vi "Motor controller.vi"() -> ()   [LabVIEW 2012]
uses:
  BotStatus.vi
  <vilib>/Rock Robotics/WPI/Solenoid/WPI_SolenoidSetEnum.vi
  <vilib>/Rock Robotics/WPI/Solenoid/WPI_SolenoidValue.ctl
panel:
  out "Transferable":bool
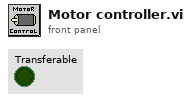
[diagram p1: front panel]
types:
  T1 = typedef "WPI_SolenoidValue.ctl" = enum16{"Off", "On", "Forward", "Reverse"}
  T2 = typedef "WPI_MotorControlDeviceRef.ctl" = cluster{"DeviceStatus":errorcluster, "Type":enum16{"PWM", "CAN"}, "PWM":cluster{"Digital Module":T3, "PWM Channel":T4, "DeadBand":T5}, "CAN":cluster{"Device Number":u8, "Control Mode":T6, "Semaphore":T7, "Max Vout":dbl}, "Invert":bool, "TransformRef":T8, "InvTransformRef":T8}
  T3 = typedef "FPGA_TypedefDigitalModule.ctl" = enum16{"Digital Module 1", "Digital Module 2"}
  T4 = typedef "FPGA_DIOPWMChannel.ctl" = enum8{"PWM 1", "PWM 2", "PWM 3", "PWM 4", "PWM 5", "PWM 6", "PWM 7", "PWM 8", "PWM 9", "PWM 10", "Invalid"}
  T5 = typedef "WPI_PWMDeadband.ctl" = cluster{"Name":string, "maxPositivePwm":i32, "minPositivePwm":i32, "centerPwm":i32, "maxNegativePwm":i32, "minNegativePwm":i32, "angularRange":u16}
  T6 = typedef "WPI_CANJaguar_ControlMode.ctl" = enum8{"Percent VBus", "Current", "Speed", "Position", "Voltage"}
  T7 = typedef "Semaphore RefNum" = refnum<k1>
  T8 = typedef "WPI_PWMTransform_ConPane.ctl" = refnum<vi>
  T9 = typedef "WPI_EncoderDevRef.ctl" = cluster{"DevStatus":errorcluster, "EncoderIndex":T10, "CounterIndex":T11, "DistancePerCount":dbl, "Decoding Type":T12}
  T10 = typedef "FPGA_EncoderIdx.ctl" = enum8{"Enc 0", "Enc 1", "Enc 2", "Enc 3", "Invalid"}
  T11 = typedef "FPGA_CounterCtrSystemIndex.ctl" = enum8{"Ctr 0", "Ctr 1", "Ctr 2", "Ctr 3", "Ctr 4", "Ctr 5", "Ctr 6", "Ctr 7", "Invalid"}
  T12 = typedef "WPI_EncoderType.ctl" = enum16{"1x", "2x", "4x"}
  T13 = typedef "WPI_RelayDevRef.ctl" = cluster{"DevStatus":errorcluster, "Relay Channel":T14, "Digital Module":T3, "Relay Direction":T15}
  T14 = typedef "FPGA_DIORelayChannel.ctl" = enum8{"Relay 1", "Relay 2", "Relay 3", "Relay 4", "Relay 5", "Relay 6", "Relay 7", "Relay 8", "Invalid"}
  T15 = typedef "WPI_RelayDirection.ctl" = enum16{"Both directions", "Forward only", "Reverse only"}
  T16 = typedef "WPI_RelayValue.ctl" = enum16{"Off", "On", "Forward", "Reverse"}
  T17 = typedef "WPI_ServoDeviceRef.ctl" = cluster{"DeviceStatus":errorcluster, "Digital Module":T3, "PWM Channel":T4, "DeadBand":T5}
  T18 = typedef "WPI_SolenoidDevRef.ctl" = cluster{"DevStatus":errorcluster, "Solenoid Module":T19, "Forward Solenoid Channel":T20, "Reverse Solenoid Channel":T20}
  T19 = typedef "FPGA_TypedefSolenoidModule.ctl" = enum16{"Solenoid Module 1", "Solenoid Module 2"}
  T20 = typedef "WPI_SolenoidChannel.ctl" = enum8{"Solenoid 1", "Solenoid 2", "Solenoid 3", "Solenoid 4", "Solenoid 5", "Solenoid 6", "Solenoid 7", "Solenoid 8", "Invalid"}
  T21 = cluster{"Cannon Upper LS":bool, "Cannon Lower LS":bool}
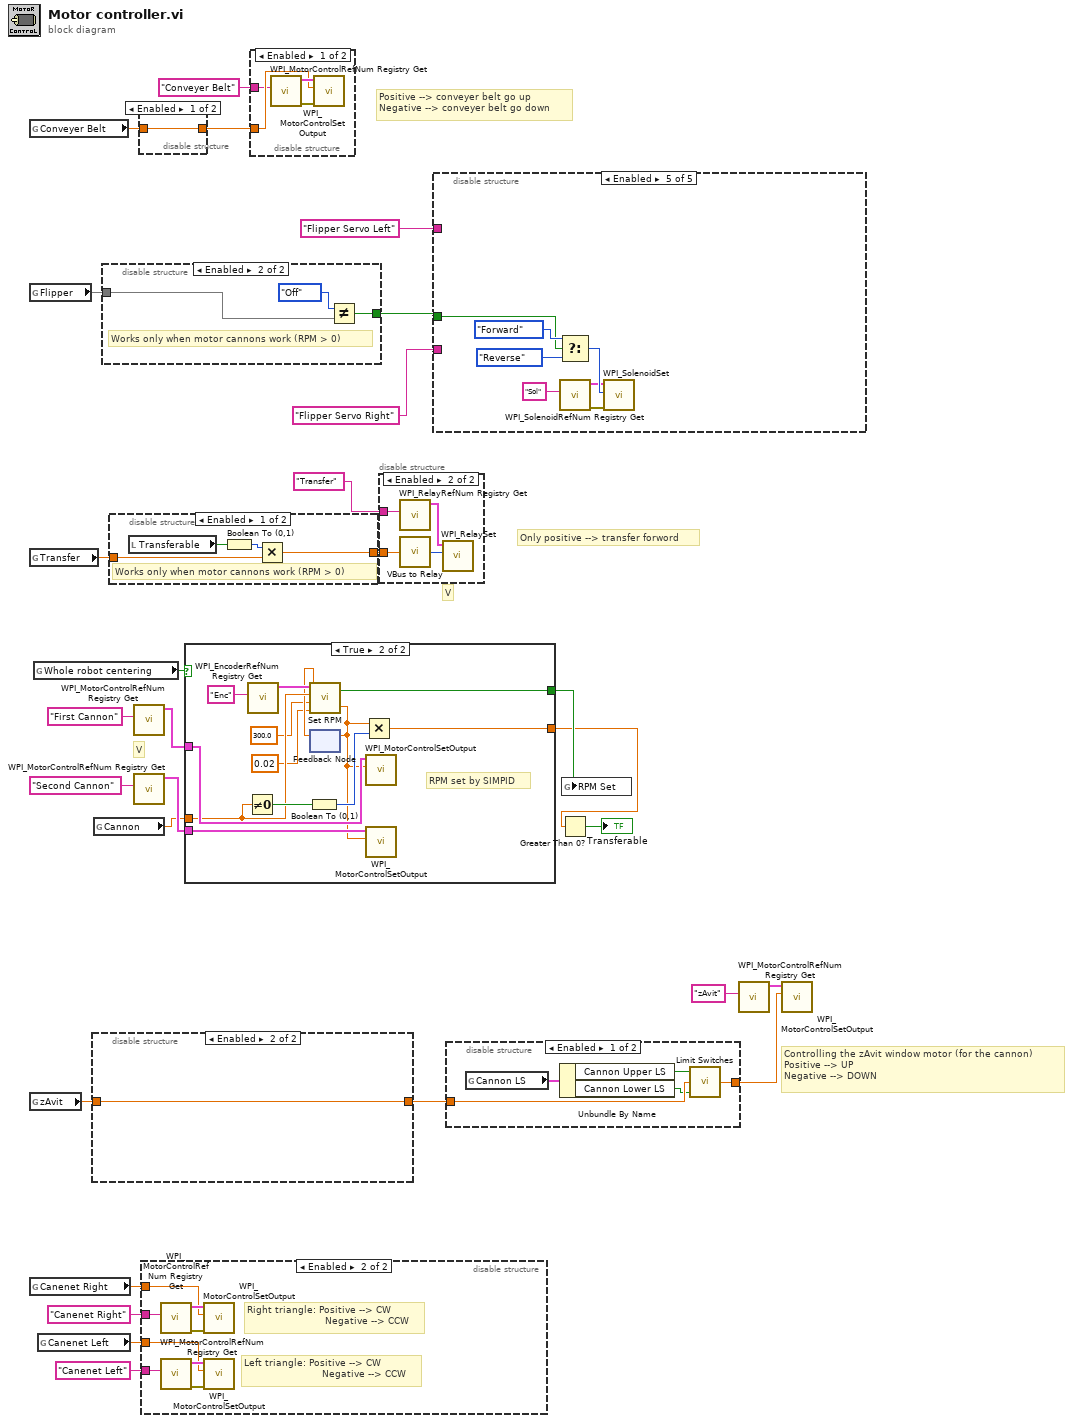
[diagram p0: block diagram]
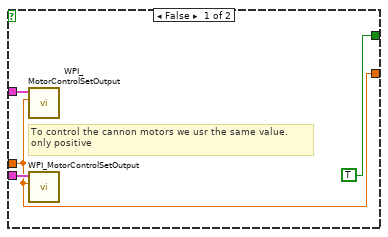
[diagram p2: hidden frame]
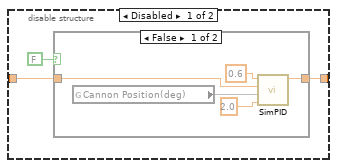
[diagram p4: hidden frame]
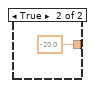
[diagram p5: hidden frame]
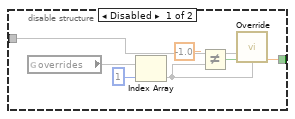
[diagram p8: hidden frame]
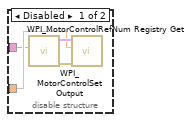
[diagram p10: hidden frame]
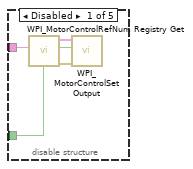
[diagram p11: hidden frame]
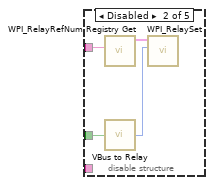
[diagram p12: hidden frame]
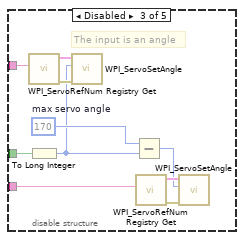
[diagram p13: hidden frame]
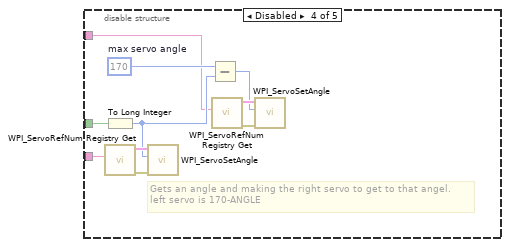
[diagram p14: hidden frame]
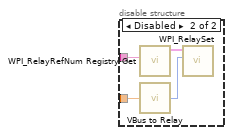
[diagram p15: hidden frame]
diagram:
  # "Positive --> conveyer belt go up\nNegative --> conveyer belt go down"
  # "Only positive --> transfer forword"
  # "Controlling the zAvit window motor (for the cannon)\nPositive --> UP\nNegative --> DOWN"
  # "V"
  # "V"
  n1 = global read "BotStatus.vi" "Conveyer Belt"() -> (w12:dbl)
  n2 = global read "BotStatus.vi" "Flipper"() -> (w13)
  n3 = global read "BotStatus.vi" "Transfer"() -> (w14:dbl)
  n4 = global read "BotStatus.vi" "zAvit"() -> (w15:dbl)
  n5 = global read "BotStatus.vi" "Canenet Right"() -> (w10:dbl)
  n6 = global read "BotStatus.vi" "Whole robot centering"() -> (w1:bool)
  n7 = global read "BotStatus.vi" "Canenet Left"() -> (w11:dbl)
  n8 = disable-structure shown="Enabled" {
    disable-tunnel: [w31 w38] -> w17
    disable-tunnel: w15 -> [w30 w38]
    frame Disabled {
      n9 = case shown="False" FALSE {
        tunnel: [w32 -20.0 ("zAvit")] -> w31
        tunnel: w30 -> [w36 _]
        frame False {
          n10 = global read "BotStatus.vi" "Cannon Position(deg)"() -> (w35)
          n11 = call "SimPID.vi"("Range"=2.0, "Position"=w35, "Set Point"=w36, "Gain"=0.6) -> ("result"=w32:dbl)  [unwired: 5 in, 1 out]
        }
        frame True {
        }
      }
    }
    frame Enabled {
    }
  }
  n12 = global read "BotStatus.vi" "Cannon"() -> (w3:dbl)
  n13 = disable-structure shown="Enabled" {
    disable-tunnel: w13 -> [w45 w48]
    disable-tunnel: [w44 w47] -> w19
    frame Disabled {
      n14 = global read "BotStatus.vi" "overrides"() -> (w43)
      n15 = Index Array(array=w43, index=1) -> (element=w39)
      n16 = Not Equal?(x=-1.0, y=w39) -> (x != y?=w40:bool)
      n17 = call "Override.vi"("Regualer"=w45, "Override"=w40, "Overriden"=w39) -> ("Output"=w44:dbl)  [unwired: 12 in]
    }
    frame Enabled {
      # "Works only when motor cannons work (RPM > 0)"
      n18 = Not Equal?(x=WPI_SolenoidValue."Off" ("Value"), y=w48) -> (x != y?=w47:bool)
    }
  }
  n19 = disable-structure shown="Enabled" {
    disable-tunnel: w14 -> [w52 w53]
    disable-tunnel: [w49 w53] -> w18
    frame Enabled {
      # "Works only when motor cannons work (RPM > 0)"
      n20 = local read "Transferable"() -> (w51:bool)
      n21 = Boolean To (0,1)(Boolean=w51) -> (0, 1=w50:i16)
      n22 = Multiply(x=w50, y=w52) -> (x*y=w49:dbl)
    }
    frame Disabled {
    }
  }
  n23 = call <vilib>:"WPI_MotorControlRefNum Registry Get.vi"("refnum name"="First Cannon") -> ("MotorControlDevRef"=w7:T2)  [unwired: 9 in, 1 out]
  n24 = call <vilib>:"WPI_MotorControlRefNum Registry Get.vi"("refnum name"="Second Cannon") -> ("MotorControlDevRef"=w6:T2)  [unwired: 9 in, 1 out]
  n25 = disable-structure shown="Enabled" {
    disable-tunnel: [w54 w55] -> w20
    disable-tunnel: w12 -> [w54 w55]
    frame Enabled {
    }
    frame Disabled {
    }
  }
  n26 = disable-structure shown="Enabled" {
    disable-tunnel: "Canenet Right" ("refnum name") -> [_ w59]
    disable-tunnel: "Canenet Left" ("refnum name") -> [_ w58]
    disable-tunnel: w10 -> [_ w57]
    disable-tunnel: w11 -> [_ w56]
    frame Disabled {
    }
    frame Enabled {
      # "Left triangle: Positive --> CW\n                          Negative --> CCW"
      # "Right triangle: Positive --> CW\n                          Negative --> CCW"
      n27 = call <vilib>:"WPI_MotorControlRefNum Registry Get.vi"("refnum name"=w59) -> ("error out"=w63:errorcluster, "MotorControlDevRef"=w62:T2)  [unwired: 9 in]
      n28 = call <vilib>:"WPI_MotorControlRefNum Registry Get.vi"("refnum name"=w58) -> ("error out"=w60:errorcluster, "MotorControlDevRef"=w61:T2)  [unwired: 9 in]
      n29 = call <vilib>:"WPI_MotorControlSetOutput.vi"("error in (no error)"=w63, "Output"=w57, "MotorControlDevRef"=w62) -> ()  [unwired: 6 in, 3 out]
      n30 = call <vilib>:"WPI_MotorControlSetOutput.vi"("error in (no error)"=w60, "Output"=w56, "MotorControlDevRef"=w61) -> ()  [unwired: 6 in, 3 out]
    }
  }
  n31 = case shown="True" w1 {
    tunnel: w7 -> [w67 w76]
    tunnel: w6 -> [w66 w75]
    tunnel: [TRUE w74] -> w4
    tunnel: w3 -> [w64 w72]
    tunnel: [w64 w73] -> w2
    frame False {
      # "To control the cannon motors we usr the same value.\nonly positive"
      n32 = call <vilib>:"WPI_MotorControlSetOutput.vi"("Output"=w64, "MotorControlDevRef"=w67) -> ()  [unwired: 7 in, 3 out]
      n33 = call <vilib>:"WPI_MotorControlSetOutput.vi"("Output"=w64, "MotorControlDevRef"=w66) -> ()  [unwired: 7 in, 3 out]
    }
    frame True {
      # "RPM set by SIMPID"
      n34 = Not Equal To 0?(x=w72) -> (x != 0?=w78:bool)
      n35 = call <vilib>:"WPI_EncoderRefNum Registry Get.vi"("refnum name"="Enc") -> ("EncoderDevRef"=w79:T9)  [unwired: 9 in, 1 out]
      n36 = Boolean To (0,1)(Boolean=w78) -> (0, 1=w77:i16)
      n37 = feedback #1() -> (w70:dbl)  [unwired: 1 in]
      n38 = call "Set RPM.vi"("EncoderDevRef"=w79, "Set Point RPM"=w72, "Range RPM"=300.0, "Gain Vbus"=0.02, "Previous Vbus"=w70) -> ("READY!"=w74:bool, "Vbus Out"=w71:dbl)
      n39 = feedback-in #1(w71) -> ()
      n40 = Multiply(x=w71, y=w77) -> (x*y=w73:dbl)
      n41 = call <vilib>:"WPI_MotorControlSetOutput.vi"("Output"=w71, "MotorControlDevRef"=w76) -> ()  [unwired: 7 in, 3 out]
      n42 = call <vilib>:"WPI_MotorControlSetOutput.vi"("Output"=w71, "MotorControlDevRef"=w75) -> ()  [unwired: 7 in, 3 out]
    }
  }
  n43 = disable-structure shown="Enabled" {
    disable-tunnel: w20 -> [w82 w85]
    disable-tunnel: "Conveyer Belt" ("refnum name") -> [w81 w87]
    frame Enabled {
      n44 = call <vilib>:"WPI_MotorControlRefNum Registry Get.vi"("refnum name"=w81) -> ("error out"=w84:errorcluster, "MotorControlDevRef"=w83:T2)  [unwired: 9 in]
      n45 = call <vilib>:"WPI_MotorControlSetOutput.vi"("error in (no error)"=w84, "Output"=w82, "MotorControlDevRef"=w83) -> ()  [unwired: 6 in, 3 out]
    }
    frame Disabled {
      n46 = call <vilib>:"WPI_RelayRefNum Registry Get.vi"("refnum name"=w87) -> ("RelayDevRef"=w86:T13)  [unwired: 9 in, 1 out]
      n47 = call "VBus to Relay.vi"("Motor VBus"=w85) -> ("RelayValue"=w88:T16)  [unwired: 3 in]
      n48 = call <vilib>:"WPI_RelaySet.vi"("RelayValue"=w88, "RelayDevRef"=w86) -> ()  [unwired: 8 in, 2 out]
    }
  }
  n49 = disable-structure shown="Enabled" {
    disable-tunnel: w18 -> [w90 w93]
    disable-tunnel: "Transfer" ("refnum name") -> [w89 w95]
    frame Disabled {
      n50 = call <vilib>:"WPI_MotorControlRefNum Registry Get.vi"("refnum name"=w89) -> ("error out"=w92:errorcluster, "MotorControlDevRef"=w91:T2)  [unwired: 9 in]
      n51 = call <vilib>:"WPI_MotorControlSetOutput.vi"("error in (no error)"=w92, "Output"=w90, "MotorControlDevRef"=w91) -> ()  [unwired: 6 in, 3 out]
    }
    frame Enabled {
      n52 = call <vilib>:"WPI_RelayRefNum Registry Get.vi"("refnum name"=w95) -> ("RelayDevRef"=w94:T13)  [unwired: 9 in, 1 out]
      n53 = call "VBus to Relay.vi"("Motor VBus"=w93) -> ("RelayValue"=w96:T16)  [unwired: 3 in]
      n54 = call <vilib>:"WPI_RelaySet.vi"("RelayValue"=w96, "RelayDevRef"=w94) -> ()  [unwired: 8 in, 2 out]
    }
  }
  n55 = disable-structure shown="Enabled" {
    disable-tunnel: w19 -> [w98 w101 w111 w122 w126]
    disable-tunnel: "Flipper Servo Left" ("refnum name") -> [w97 w103 w114 w116 _]
    disable-tunnel: "Flipper Servo Right" ("refnum name") -> [_ _ w105 w115 _]
    frame Disabled {
      n56 = call <vilib>:"WPI_MotorControlRefNum Registry Get.vi"("refnum name"=w97) -> ("error out"=w100:errorcluster, "MotorControlDevRef"=w99:T2)  [unwired: 9 in]
      n57 = call <vilib>:"WPI_MotorControlSetOutput.vi"("error in (no error)"=w100, "Output"=w98, "MotorControlDevRef"=w99) -> ()  [unwired: 6 in, 3 out]
    }
    frame Disabled {
      n58 = call <vilib>:"WPI_RelayRefNum Registry Get.vi"("refnum name"=w103) -> ("RelayDevRef"=w102:T13)  [unwired: 9 in, 1 out]
      n59 = call "VBus to Relay.vi"("Motor VBus"=w101) -> ("RelayValue"=w104:T16)  [unwired: 3 in]
      n60 = call <vilib>:"WPI_RelaySet.vi"("RelayValue"=w104, "RelayDevRef"=w102) -> ()  [unwired: 8 in, 2 out]
    }
    frame Disabled {
      w108 = 170  # max servo angle
      # "The input is an angle"
      n61 = call <vilib>:"WPI_ServoRefNum Registry Get.vi"("refnum name"=w114) -> ("error out"=w112:errorcluster, "ServoDeviceRef"=w113:T17)  [unwired: 9 in]
      n62 = To Long Integer(number=w111) -> (32bit integer=w107:i32)
      n63 = call <vilib>:"WPI_ServoSetAngle.vi"("error in (no error)"=w112, "Angle"=w107, "ServoDeviceRef"=w113) -> ()  [unwired: 7 in, 2 out]
      n64 = Subtract(x=w108, y=w107) -> (x-y=w106:i32)
      n65 = call <vilib>:"WPI_ServoRefNum Registry Get.vi"("refnum name"=w105) -> ("error out"=w110:errorcluster, "ServoDeviceRef"=w109:T17)  [unwired: 9 in]
      n66 = call <vilib>:"WPI_ServoSetAngle.vi"("error in (no error)"=w110, "Angle"=w106, "ServoDeviceRef"=w109) -> ()  [unwired: 7 in, 2 out]
    }
    frame Disabled {
      w119 = 170  # max servo angle
      # "Gets an angle and making the right servo to get to that angel.\nleft servo is 170-ANGLE"
      n67 = To Long Integer(number=w122) -> (32bit integer=w118:i32)
      n68 = call <vilib>:"WPI_ServoRefNum Registry Get.vi"("refnum name"=w115) -> ("error out"=w123:errorcluster, "ServoDeviceRef"=w124:T17)  [unwired: 9 in]
      n69 = call <vilib>:"WPI_ServoSetAngle.vi"("error in (no error)"=w123, "Angle"=w118, "ServoDeviceRef"=w124) -> ()  [unwired: 7 in, 2 out]
      n70 = Subtract(x=w119, y=w118) -> (x-y=w117:i32)
      n71 = call <vilib>:"WPI_ServoRefNum Registry Get.vi"("refnum name"=w116) -> ("error out"=w121:errorcluster, "ServoDeviceRef"=w120:T17)  [unwired: 9 in]
      n72 = call <vilib>:"WPI_ServoSetAngle.vi"("error in (no error)"=w121, "Angle"=w117, "ServoDeviceRef"=w120) -> ()  [unwired: 7 in, 2 out]
    }
    frame Enabled {
      n73 = Select(t=WPI_SolenoidValue."Forward" ("Value"), s=w126, f=WPI_SolenoidValue."Reverse" ("Value")) -> (s? t:f=w127:T1)
      n74 = call <vilib>:"WPI_SolenoidRefNum Registry Get.vi"("refnum name"="Sol") -> ("error out"=w130:errorcluster, "SolenoidDevRef"=w125:T18)  [unwired: 9 in]
      n75 = call-poly <vilib>:"WPI_SolenoidSet.vi"("error in (no error)"=w130, "Value"=w127, "SolenoidDevRef"=w125) -> ()  [unwired: 9 out]
    }
  }
  n76 = disable-structure shown="Enabled" {
    disable-tunnel: w17 -> [w136 w137]
    disable-tunnel: [w135 w137] -> w16
    frame Enabled {
      n77 = global read "BotStatus.vi" "Cannon LS"() -> (w132:T21)
      n78 = Unbundle By Name(w132) -> ("Cannon Upper LS"=w134:bool, "Cannon Lower LS"=w133:bool)
      n79 = call "Limit Switches.vi"("Backward Limit Switch"=w133, "VBus in"=w136, "Forward Limit Switch"=w134) -> ("VBus out"=w135:dbl)
    }
    frame Disabled {
    }
  }
  n80 = Greater Than 0?(x=w2) -> (x > 0?=→"Transferable":bool)
  n81 = global write "BotStatus.vi" "RPM Set"(w4) -> ()
  n82 = call <vilib>:"WPI_MotorControlRefNum Registry Get.vi"("refnum name"="zAvit") -> ("MotorControlDevRef"=w22:T2)  [unwired: 9 in, 1 out]
  n83 = call <vilib>:"WPI_MotorControlSetOutput.vi"("Output"=w16, "MotorControlDevRef"=w22) -> ()  [unwired: 7 in, 3 out]
